vi "HH_Histogram.vi"(0 "Data In":u32[](array[numeric])) -> (4 "Histogram":i32[](array[numeric]))   [LabVIEW 2009]
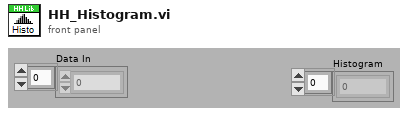
[diagram p1: front panel]
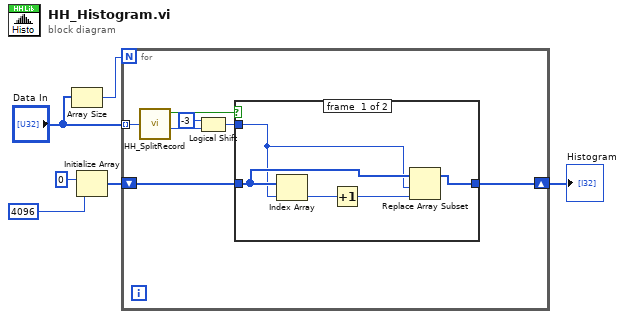
[diagram p0: block diagram]
diagram:
  n1 = Array Size(array="Data In") -> (size(s)=w1:i32)
  n2 = Initialize Array(0 ("element"), 4096 ("dimension size")) -> (w4:i32[])
  n3 = for {
    N: w1 -> [_]
    tunnel: "Data In" -> [w11] mode=indexing
    shift-right: [w12] -> w3
    shift-left: w4 -> [w13]
    n4 = call "HH_SplitRecord.vi"("Record in"=w11) -> ("Special"=w10:bool, "time"=w8:i32)  [unwired: 2 out]
    n5 = Logical Shift(y=i8 -3, x=w8) -> (x << y=w7:i32)
    n6 = case shown="False" w10 {
      tunnel: w13 -> [w17 w19]
      tunnel: [w15 w19] -> w12
      tunnel: w7 -> [w14 _]
      frame #0 {
        n7 = Index Array(array=w17, index=w14) -> (element=w18:i32)
        n8 = Increment(x=w18) -> (x+1=w16:i32)
        n9 = Replace Array Subset(array=w17, new element=w16, index=w14) -> (w15:i32[])
      }
      frame #1 {
      }
    }
  }
  "Histogram" <- w3
